vi "Current Time Strings.vi"() -> (0 "Minutes":string, 1 "Hour":string, 2 "Day":string, 3 "Month":string, 4 "Seconds":string, 5 "Year":string)   [LabVIEW 2018]
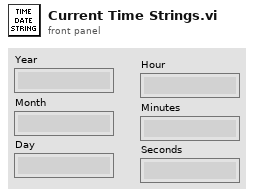
[diagram p1: front panel]
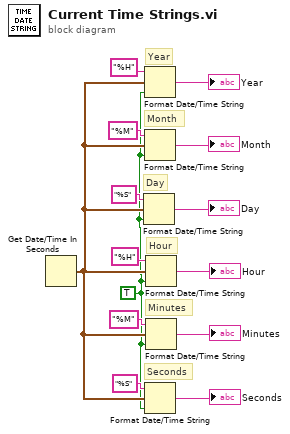
[diagram p0: block diagram]
diagram:
  w1 = TRUE ("UTC format")
  # "Day"
  # "Month"
  # "Year"
  # "Seconds"
  # "Minutes"
  # "Hour"
  n1 = Get Date/Time In Seconds() -> (seconds since 1Jan1904=w2:timestamp)
  n2 = Format Date/Time String(time format string (%c)="%S", seconds (now)=w2, UTC format=w1) -> (date/time string=→"Day":string)
  n3 = Format Date/Time String(time format string (%c)="%H", seconds (now)=w2, UTC format=w1) -> (date/time string=→"Year":string)
  n4 = Format Date/Time String(time format string (%c)="%M", seconds (now)=w2, UTC format=w1) -> (date/time string=→"Month":string)
  n5 = Format Date/Time String(time format string (%c)="%S", seconds (now)=w2, UTC format=w1) -> (date/time string=→"Seconds":string)
  n6 = Format Date/Time String(time format string (%c)="%H", seconds (now)=w2, UTC format=w1) -> (date/time string=→"Hour":string)
  n7 = Format Date/Time String(time format string (%c)="%M", seconds (now)=w2, UTC format=w1) -> (date/time string=→"Minutes":string)
